vi "Enable Create Station.vi"(8 "error in (no error)":errorcluster, 11 "PLC Sim Controller Actor in":refnum<class "PLC Sim Controller Actor.lvclass">) -> (0 "error out":errorcluster, 3 "PLC Sim Controller Actor out":refnum<class "PLC Sim Controller Actor.lvclass">)   [LabVIEW 2019, in "PLC Sim Controller Actor.lvlib" / "PLC Sim Controller Actor.lvclass"]
uses:
  PLC Sim Controller Actor.lvclass
  PLC Sim Controller Actor.lvclass/PLC Sim Controller Actor.ctl
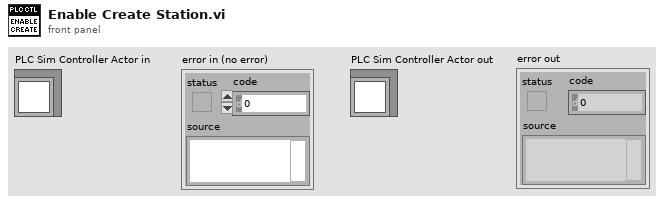
[diagram p1: front panel]
types:
  T1 = enum8{"Enabled", "Disabled", "Disabled and Grayed Out"}
  T2 = typedef "LVComboBoxStrsAndValuesArrayTypeDef.ctl" = cluster{"String":string, "Value":string}[]
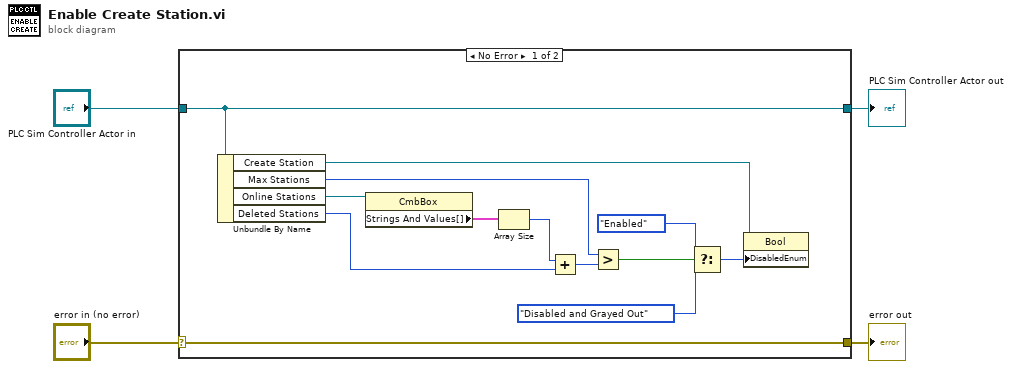
[diagram p0: block diagram]
diagram:
  n1 = case shown="No Error" "error in (no error)" {
    selector: "error in (no error)" -> [w17 w19]
    tunnel: [w17 w19] -> w3
    tunnel: [w16 w18] -> w1
    tunnel: "PLC Sim Controller Actor in" -> [w16 w18]
    frame No Error {
      n2 = Unbundle By Name(w16) -> ("Create Station"=w15:refnum<vi>, "Max Stations"=w8:i32, "Online Stations"=w7:refnum<vi>, "Deleted Stations"=w6:u32)
      n3 = property class="CmbBox"(reference=w7) -> ("Strings And Values[]"=w11:T2)  [unwired: 1 in, 2 out]
      n4 = Array Size(array=w11) -> (size(s)=w10:i32)
      n5 = Add(x=w10, y=w6) -> (x+y=w9:u32)
      n6 = Greater?(x=w8, y=w9) -> (0:w5:bool)
      n7 = Select(t=T1."Enabled" ("Disabled"), s=w5, f=T1."Disabled and Grayed Out" ("Disabled")) -> (s? t:f=w12:T1)
      n8 = property class="Bool"(reference=w15, "DisabledEnum"=w12) -> ()  [unwired: 1 in, 2 out]
    }
    frame Error {
    }
  }
  "error out" <- w3
  "PLC Sim Controller Actor out" <- w1
